vi "Detect Part Number.vi"(10 "Digit Array":T1[](array[typedef]), 11 "Unsigned Byte Array":u8[][](array[numeric])) -> (3 "Is a part Number":bool)   [LabVIEW 2023]
uses:
  Cluster Digit.ctl
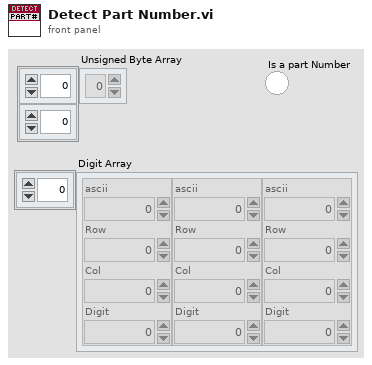
[diagram p1: front panel]
types:
  T1 = typedef "Cluster Digit.ctl" = cluster{"ascii":u8, "Row":i32, "Col":i32, "Digit":i32}
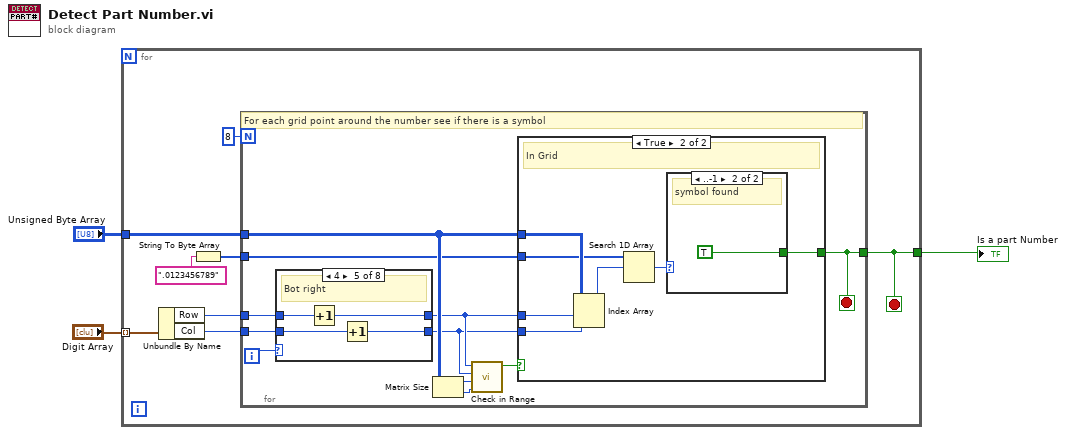
[diagram p0: block diagram]
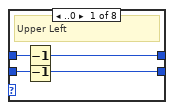
[diagram p2: hidden frame]
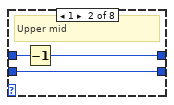
[diagram p3: hidden frame]
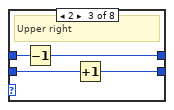
[diagram p4: hidden frame]
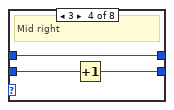
[diagram p5: hidden frame]
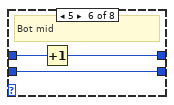
[diagram p6: hidden frame]
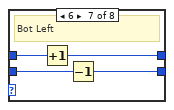
[diagram p7: hidden frame]
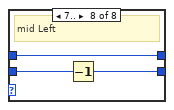
[diagram p8: hidden frame]
diagram:
  n1 = for {
    tunnel: "Digit Array" -> [w11] mode=indexing
    tunnel: "Unsigned Byte Array" -> [w9]
    tunnel: [w4] -> w3
    stop <- w4 stop-if-true
    n2 = Unbundle By Name(w11) -> ("Row"=w8:i32, "Col"=w7:i32)
    n3 = String To Byte Array(string=".0123456789" ("String")) -> (unsigned byte array=w6:u8[])
    n4 = for {
      N: 8 -> [_]
      tunnel: w6 -> [w13]
      tunnel: w9 -> [w20]
      tunnel: w8 -> [w22]
      tunnel: w7 -> [w21]
      tunnel: [w12] -> w4
      i -> [w14]
      stop <- w12 stop-if-true
      # "For each grid point around the number see if there is a symbol"
      n5 = case shown="4" w14 {
        tunnel: w22 -> [w26 w29 w33 w34 w38 w43 w47 w48]
        tunnel: w21 -> [w25 w27 w31 w36 w40 w41 w45 w50]
        tunnel: [w24 w28 w32 w34 w37 w42 w46 w48] -> w18
        tunnel: [w23 w27 w30 w35 w39 w41 w44 w49] -> w16
        frame ..0 {
          # "Upper Left"
          n6 = Decrement(x=w26) -> (x-1=w24:i32)
          n7 = Decrement(x=w25) -> (x-1=w23:i32)
        }
        frame 1 {
          # "Upper mid"
          n8 = Decrement(x=w29) -> (x-1=w28:i32)
        }
        frame 2 {
          # "Upper right"
          n9 = Decrement(x=w33) -> (x-1=w32:i32)
          n10 = Increment(x=w31) -> (x+1=w30:i32)
        }
        frame 3 {
          # "Mid right"
          n11 = Increment(x=w36) -> (x+1=w35:i32)
        }
        frame 4 {
          # "Bot right"
          n12 = Increment(x=w38) -> (x+1=w37:i32)
          n13 = Increment(x=w40) -> (x+1=w39:i32)
        }
        frame 5 {
          # "Bot mid"
          n14 = Increment(x=w43) -> (x+1=w42:i32)
        }
        frame 6 {
          # "Bot Left"
          n15 = Increment(x=w47) -> (x+1=w46:i32)
          n16 = Decrement(x=w45) -> (x-1=w44:i32)
        }
        frame 7.. {
          # "mid Left"
          n17 = Decrement(x=w50) -> (x-1=w49:i32)
        }
      }
      n18 = Matrix Size(0:w20) -> (1:w17:i32, 2:w15:i32)
      n19 = call "Check in Range.vi"("number of col"=w15, "number of rows"=w17, "col"=w16, "row"=w18) -> ("in range"=w19:bool)  [unwired: 7 in]
      n20 = case shown="True" w19 {
        tunnel: w20 -> [_ w57]
        tunnel: w16 -> [_ w55]
        tunnel: w18 -> [_ w56]
        tunnel: w13 -> [_ w54]
        tunnel: [_ w51] -> w12
        frame False {
          # "Out of Grid"
        }
        frame True {
          # "In Grid"
          n21 = Index Array(array=w57, index (row)=w56, index (col)=w55) -> (element=w53:u8)
          n22 = Search 1D Array(1D array=w54, element=w53) -> (index of element=w52:i32)  [unwired: 1 in]
          n23 = case shown="..-1" w52 {
            tunnel: [_ TRUE] -> w51
            frame 0.. {
              # "Not a symbol"
            }
            frame ..-1 {
              # "symbol found"
            }
          }
        }
      }
    }
  }
  "Is a part Number" <- w3
